vi "Write Char.vi"(5 "Col":i32, 6 "Attributes":T1, 8 "error in (no error)":errorcluster, 10 "Char":string, 11 "TermLine in":refnum<class "TermLine.lvclass">) -> (0 "error out":errorcluster, 3 "TermLine out":refnum<class "TermLine.lvclass">)   [LabVIEW 2020, in "Terminal.lvlib" / "TermLine.lvclass"]
uses:
  TermLine.lvclass
  Text Attributes.ctl
  TermLine.lvclass/TermLine.ctl
  Terminal.lvlib
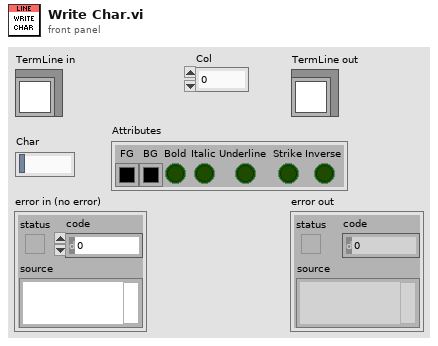
[diagram p1: front panel]
types:
  T1 = typedef "Terminal.lvlib/Text Attributes.ctl" = cluster{"FG":u32, "BG":u32, "Bold":bool, "Italic":bool, "Underline":bool, "Strike":bool, "Inverse":bool}
  T2 = typedef "Terminal.lvlib/TermLine.lvclass/Ref Data.ctl" = cluster{"Chars":T3[], "Width":i32, "Touched":bool}
  T3 = typedef "Terminal.lvlib/Term Char.ctl" = cluster{"Char":string, "Attributes":T1}
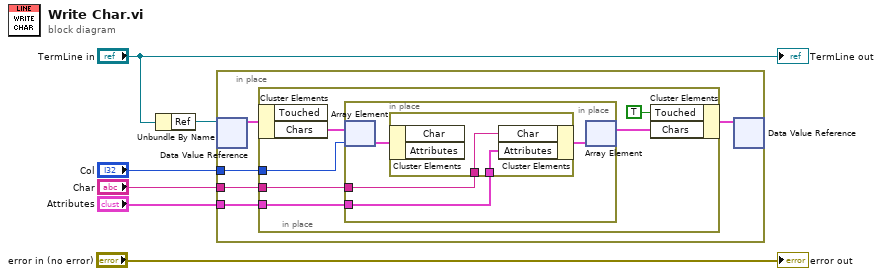
[diagram p0: block diagram]
diagram:
  n1 = Unbundle By Name("TermLine in") -> ("Ref"=w5:refnum<data-value>)
  n2 = in-place {
    in-place-border: "Col" -> [w9]
    in-place-border: "Char" -> [w8]
    in-place-border: "Attributes" -> [w7]
    n3 = in-place-dvr #1(w5) -> (w11:T2)  [unwired: 1 out]
    n4 = in-place {
      in-place-border: w9 -> [w16]
      in-place-border: w8 -> [w14]
      in-place-border: w7 -> [w13]
      n5 = in-place-cluster #2(w11) -> ("Chars"=w17:T3[])  [unwired: 1 out]
      n6 = in-place {
        in-place-border: w14 -> [w19]
        in-place-border: w13 -> [w18]
        n7 = in-place-array #3(w17, w16) -> (w21:T3)
        n8 = in-place {
          in-place-border: w19 -> [w23]
          in-place-border: w18 -> [w22]
          n9 = in-place-cluster #4(w21) -> ()  [unwired: 2 out]
          n10 = in-place-cluster #4("Char"=w23, "Attributes"=w22) -> (w20:T3)
        }
        n11 = in-place-array #3(w20) -> (w15:T3[])  [unwired: 1 out]
      }
      n12 = in-place-cluster #2("Touched"=TRUE, "Chars"=w15) -> (w10:T2)
    }
    n13 = in-place-dvr #1(w10) -> ()  [unwired: 2 out]
  }
  "error out" <- "error in (no error)"
  "TermLine out" <- "TermLine in"
